vi "Stop Core.vi"(10 "final error code":i32, 11 "Measurement_Binary in":refnum<class "Measurement_Binary.lvclass">) -> (3 "Measurement_Binary out":refnum<class "Measurement_Binary.lvclass">)   [LabVIEW 2020, in "Measurement_Binary.lvlib" / "Measurement_Binary.lvclass"]
doc: "(<B>Filename</B>: Actor Framework.lvlib:Actor.lvclass:Stop Core.vi)\n\nDefines what the actor does before it stops. Use the <B>final error code</B> input to determine whether the actor shut down in response to an error.\n\nBy default, this method passes the Stop message along to all auto-stop nested actors. A descendant class may override this method to define additional behavior, such as shutting down any processes the actor initiated in its override of the Actor Core method."
uses:
  Measurement_Binary.lvclass
  <vilib>/ActorFramework/Actor/Actor.lvclass
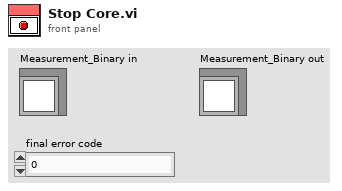
[diagram p1: front panel]
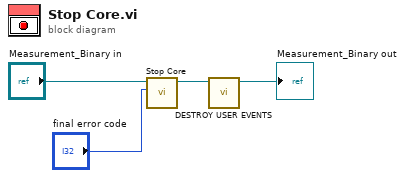
[diagram p0: block diagram]
diagram:
  n1 = call-parent "Stop Core.vi"("final error code"="final error code", "Actor in"="Measurement_Binary in") -> ("Actor out"=w2:refnum<class "Measurement_Binary.lvclass">)  [unwired: 9 in]
  n2 = call "DESTROY USER EVENTS.vi"("Measurement_Binary in"=w2) -> ("Measurement_Binary out"=→"Measurement_Binary out":refnum<class "Measurement_Binary.lvclass">)  [unwired: 9 in, 1 out]
